vi "ProdaNG.Convert.TruncZeros.vi"(11 "string with \\0s":string) -> (3 "LV string":string)   [LabVIEW 2016]
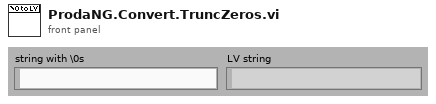
[diagram p1: front panel]
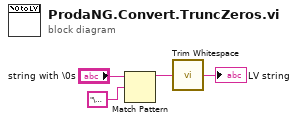
[diagram p0: block diagram]
diagram:
  n1 = Match Pattern(string="string with \\0s", regular expression="\u0000") -> (before substring=w3:string)  [unwired: 1 in, 3 out]
  n2 = call <vilib>:"Trim Whitespace.vi"("string"=w3) -> ("trimmed string"=→"LV string":string)  [unwired: 1 in]
